vi "Calc Update Rate.vi"() -> (2 "Update Rate":dbl format="%0.2f")   [LabVIEW 2020, in "FormulaG.lvlib" / "FormulaG App.lvclass"]
uses:
  FormulaG App.lvclass
  <vilib>/ptbypt/NI_PtbyPt.lvlib
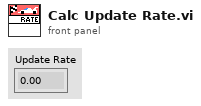
[diagram p1: front panel]
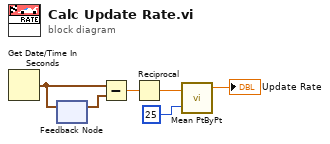
[diagram p0: block diagram]
diagram:
  n1 = Get Date/Time In Seconds() -> (seconds since 1Jan1904=w3:timestamp)
  n2 = feedback #1() -> (w4:timestamp)  [unwired: 1 in]
  n3 = feedback-in #1(w3) -> ()
  n4 = Subtract(x=w3, y=w4) -> (x-y=w5:dbl)
  n5 = Reciprocal(x=w5) -> (1/x=w6:dbl)
  n6 = call <vilib>:"Mean PtByPt.vi"("x"=w6, "sample length"=25) -> ("mean"=→"Update Rate":dbl)  [unwired: 2 in, 1 out]
